vi "Handle.vi"(8 "error in (no error)":errorcluster, 11 "Publisher in":refnum<class "Publisher.lvclass">) -> (0 "error out":errorcluster, 3 "Publisher out":refnum<class "Publisher.lvclass">)   [LabVIEW 2018, in "Publisher.lvclass"]
uses:
  Publisher.lvclass
  Publisher.lvclass/Publisher.ctl
  Client/Client.lvclass
  Comm/Stream/Stream.lvclass
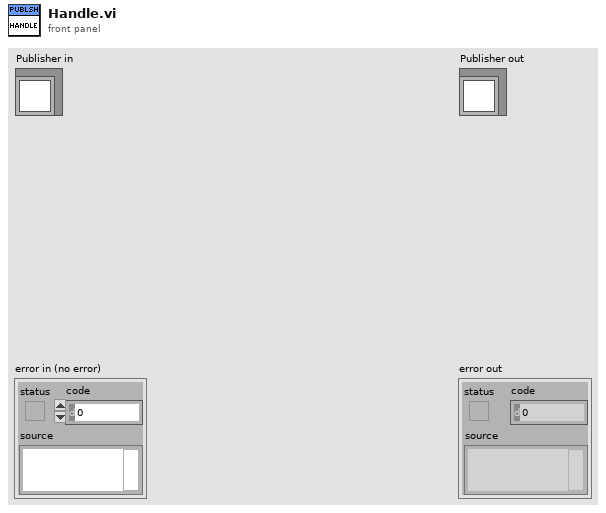
[diagram p1: front panel]
types:
  T1 = cluster{"OBSERVER":string, "OBJECT":string, "CTRLINTE":string, "PROJID":string, "SYNCMODE":string, "INSTMODE":string, "FILTER":string, "OBSTYPE":string, "CHANNEL 1":bool, "CHANNEL 2":bool, "CHANNEL 3":bool, "CHANNEL 4":bool, "TCSMODE":bool, "COMMENT":string, "BROKER":string}
  T2 = cluster{"OBSERVER":string, "OBJECT":string, "CTRLINTE":string, "PROJID":string, "SYNCMODE":string, "INSTMODE":string, "FILRTER":string, "OBSTYPE":string, "CHANNEL 1":bool, "CHANNEL 2":bool, "CHANNEL 3":bool, "CHANNEL 4":bool, "TCSMODE":bool, "COMMENT":string, "BROKER":string}
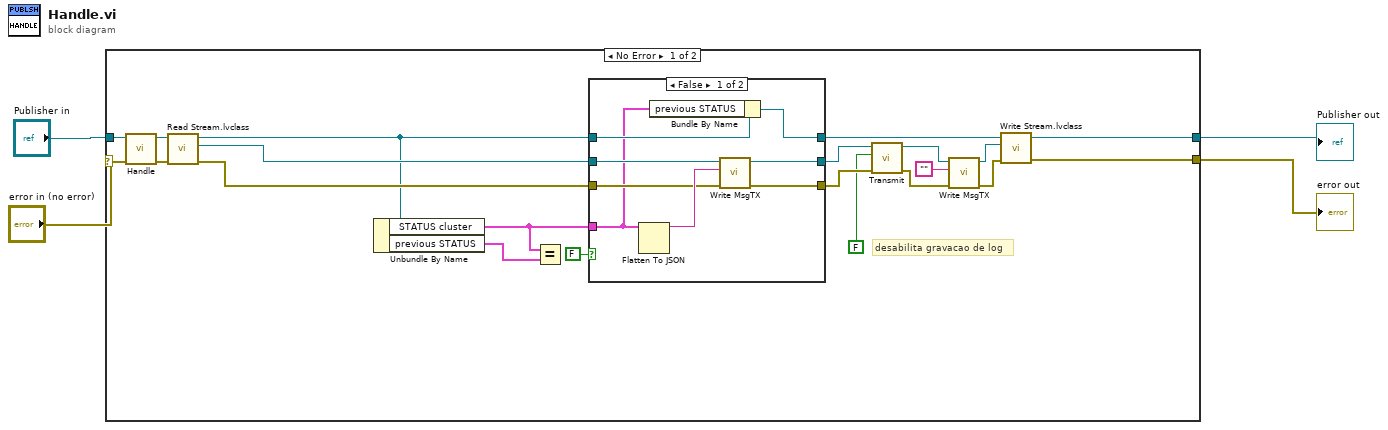
[diagram p0: block diagram]
diagram:
  n1 = call-parent "Handle.vi"("error in (no error)"="error in (no error)", "Client in"="Publisher in") -> ("error out"=w3:errorcluster, "Client out"=w4:refnum<class "Publisher.lvclass">)  [unwired: 8 in]
  n2 = case shown="No Error" w3 {
    selector: w3 -> [w24 w38]
    tunnel: [w18 w38] -> w1
    tunnel: [w19 w37] -> w2
    tunnel: w4 -> [w25 w37]
    frame No Error {
      # "desabilita gravacao de log"
      n3 = call-dynamic "Read Stream.lvclass.vi"("error in (no error)"=w24, "Client in"=w25) -> ("error out"=w17:errorcluster, "Stream.lvclass"=w20:refnum<class "Stream.lvclass">, "Client out"=w9:refnum<class "Publisher.lvclass">)  [unwired: 7 in]
      n4 = Unbundle By Name(w9) -> ("STATUS cluster"=w10:T1, "previous STATUS"=w16:T2)
      n5 = Equal?(x=w10, y=w16) -> ()  [unwired: 1 out]
      n6 = case shown="False" FALSE {
        tunnel: [w33 w36] -> w23
        tunnel: [w32 w35] -> w22
        tunnel: w20 -> [w31 w36]
        tunnel: w17 -> [w29 w35]
        tunnel: w10 -> [w27 _]
        tunnel: [w26 w34] -> w8
        tunnel: w9 -> [w28 w34]
        frame False {
          n7 = Flatten To JSON(anything=w27) -> (JSON string=w30:string)  [unwired: 2 in, 1 out]
          n8 = Bundle By Name(cluster=w28, "previous STATUS"=w27) -> (w26:refnum<class "Publisher.lvclass">)
          n9 = call-dynamic "Write MsgTX.vi"("error in (no error)"=w29, "MsgTX"=w30, "Comm in"=w31) -> ("error out"=w32:errorcluster, "Comm out"=w33:refnum<class "Stream.lvclass">)  [unwired: 7 in]
        }
        frame True {
        }
      }
      n10 = call-dynamic "Transmit.vi"("error in (no error)"=w22, "log?"=FALSE, "Stream in"=w23) -> ("error out"=w14:errorcluster, "Stream out"=w15:refnum<class "Stream.lvclass">)  [unwired: 7 in]
      n11 = call-dynamic "Write MsgTX.vi"("error in (no error)"=w14, "MsgTX"="", "Comm in"=w15) -> ("error out"=w13:errorcluster, "Comm out"=w12:refnum<class "Stream.lvclass">)  [unwired: 7 in]
      n12 = call-dynamic "Write Stream.lvclass.vi"("error in (no error)"=w13, "Stream.lvclass"=w12, "Client in"=w8) -> ("error out"=w18:errorcluster, "Client out"=w19:refnum<class "Publisher.lvclass">)  [unwired: 7 in]
    }
    frame Error {
    }
  }
  "error out" <- w1
  "Publisher out" <- w2
